vi "Init.vi"(8 "error in (no error)":errorcluster, 9 "SA Pin":string, 10 "Measurement Name":string) -> (0 "error out":errorcluster, 3 "Insertion Loss out":refnum<class "Insertion Loss.lvclass">)   [LabVIEW 2016, in "SeqAuto Evaluations.lvlib" / "Insertion Loss.lvclass"]
uses:
  Insertion Loss.lvclass
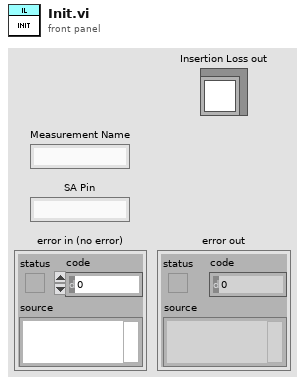
[diagram p1: front panel]
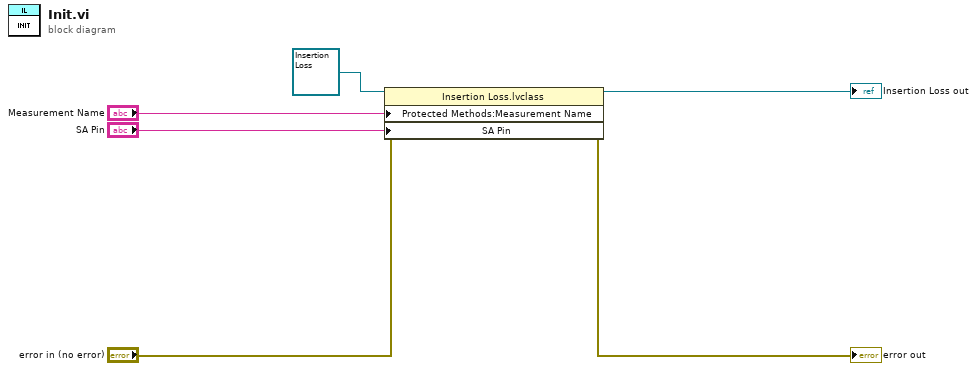
[diagram p0: block diagram]
diagram:
  n1 = property class="Insertion Loss.lvclass"(reference=refnum<class "Insertion Loss.lvclass"> refnum, error in="error in (no error)", "Protected Methods:Measurement Name"="Measurement Name", "SA Pin"="SA Pin") -> (reference out=→"Insertion Loss out":refnum<class "Insertion Loss.lvclass">, error out=→"error out":errorcluster)
